vi "set_file_sent.vi"(8 "error in (no error)":errorcluster, 10 "path array in":path[](array[path]), 11 "ErrorController in":refnum<class "ErrorController.lvclass">) -> (0 "error out":errorcluster, 3 "ErrorController out":refnum<class "ErrorController.lvclass">)   [LabVIEW 2010, in "ErrorController.lvclass"]
uses:
  ErrorController.lvclass
  <vilib>/Utility/file.llb/Write To Spreadsheet File (string).vi
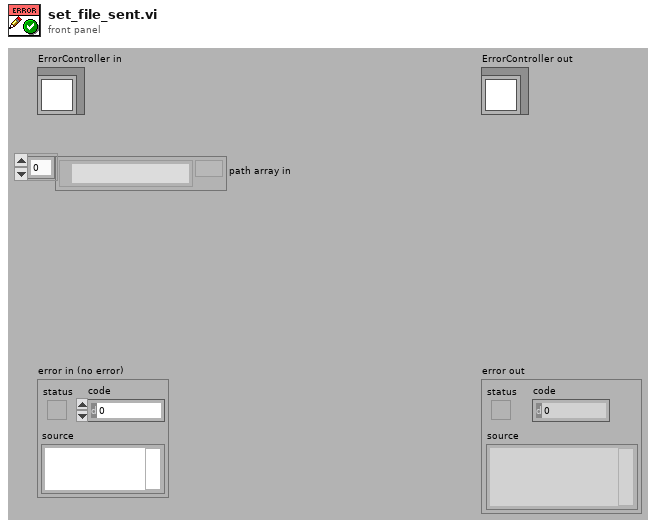
[diagram p1: front panel]
types:
  T1 = enum16{"open", "replace", "create", "open or create", "replace or create", "replace or create with confirmation"}
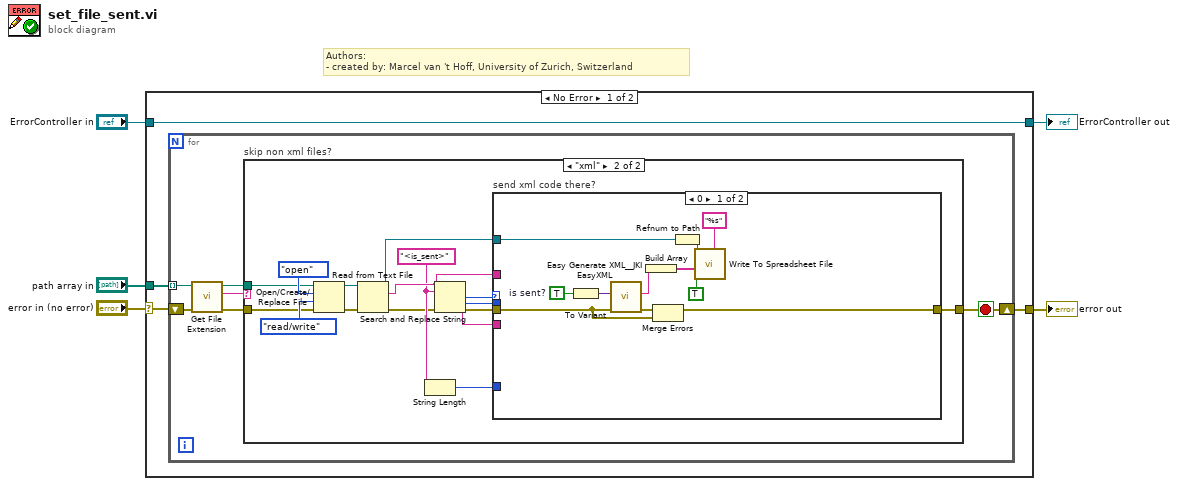
[diagram p0: block diagram]
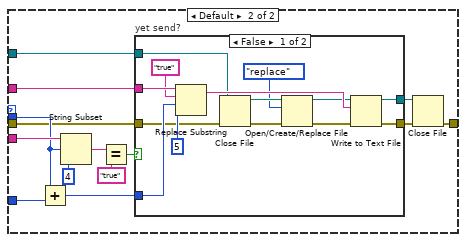
[diagram p3: hidden frame]
diagram:
  # "Authors: \n- created by: Marcel van 't Hoff, University of Zurich, Switzerland"
  n1 = case shown="No Error" "error in (no error)" {
    selector: "error in (no error)" -> [w8 w75]
    tunnel: [w7 w75] -> w4
    tunnel: [w9 w74] -> w2
    tunnel: "ErrorController in" -> [w9 w74]
    tunnel: "path array in" -> [w6 _]
    frame No Error {
      n2 = for {
        tunnel: w6 -> [w12] mode=indexing
        shift-right: [w15] -> w7
        shift-left: w8 -> [w14]
        stop <- w15 stop-if-true
        n3 = call <vilib>:"Get File Extension.vi"("error in (no error)"=w14, "file"=w12) -> ("error out"=w13:errorcluster, "lowercase file extension"=w10:string, "dup file"=w11:path)  [unwired: 6 in, 1 out]
        n4 = case "skip non xml files?" shown="\"xml\"" w10 {
          tunnel: w11 -> [_ w29]
          tunnel: w13 -> [w16 w23]
          tunnel: [w16 w19] -> w15
          frame Default {
          }
          frame "xml" {
            w26 = "<is_sent>" ("search string")
            n5 = Open/Create/Replace File(file path (use dialog)=w29, error in=w23, operation (0:open)=T1."open", access (0:read/write)=enum16{"read/write", "read-only", "write-only"}."read/write") -> (refnum out=w18:refnum<file>, error out=w30:errorcluster)  [unwired: 2 in, 1 out]
            n6 = Read from Text File(file (use dialog)=w18, error in=w30) -> (refnum out=w17:refnum<file>, text=w27:string, error out=w22:errorcluster)  [unwired: 2 in, 1 out]
            n7 = String Length(string=w26) -> (length=w25:i32)
            n8 = Search and Replace String(input string=w27, search string=w26, error in=w22) -> (result string=w28:string, number of replacements=w20:i32, offset past replacement=w24:i32, error out=w21:errorcluster)  [unwired: 5 in]
            n9 = case "send xml code there?" shown="0" w20 {
              tunnel: w28 -> [_ w53]
              tunnel: w17 -> [w37 w52]
              tunnel: w27 -> [_ w51]
              tunnel: w25 -> [_ w50]
              tunnel: w24 -> [_ w49]
              tunnel: [w33 w46] -> w19
              tunnel: w21 -> [w35 w44]
              frame 0 {
                w38 = TRUE  # is sent?
                n10 = To Variant(anything=w38) -> (Variant=w39:variant)
                n11 = call <vilib>:"Easy Generate XML__JKI EasyXML.vi"("error in (no error)"=w35, "LabVIEW Data"=w39) -> ("error out"=w34:errorcluster, "XML String"=w42:string)  [unwired: 8 in]
                n12 = Build Array(w42) -> (w43:string[])
                n13 = Merge Errors(w34, w35) -> (w33:errorcluster)
                n14 = Refnum to Path(1:w37) -> (0:w36:path)
                n15 = call-poly <vilib>:"Write To Spreadsheet File.vi"("format (%s)"="%s" ("format (%.3f)"), "append to file? (new file:F)"=TRUE, "1D data"=w43, "file path (dialog if empty)"=w36) -> ()  [unwired: 4 in, 1 out]
              }
              frame Default {
                n16 = Add(x=w49, y=w50) -> (x+y=w48:i32)
                n17 = String Subset(string=w53, offset (0)=w49, length (rest)=4 ("length (rest)")) -> (substring=w57:string)
                n18 = Equal?(x=w57, y="true") -> (x = y?=w54:bool)
                n19 = case "yet send?" shown="False" w54 {
                  tunnel: w51 -> [w69 _]
                  tunnel: w52 -> [w64 w73]
                  tunnel: w44 -> [w63 w72]
                  tunnel: [w71 w72] -> w45
                  tunnel: [w70 w73] -> w47
                  tunnel: w48 -> [w68 _]
                  frame False {
                    n20 = Replace Substring(2:5 ("length (len. of substring)"), 3:w68, 4:"true" ("replace string (\"\")"), 5:w69) -> (1:w65:string)  [unwired: 1 out]
                    n21 = Close File(refnum=w64, error in=w63) -> (path=w62:path, error out=w61:errorcluster)
                    n22 = Open/Create/Replace File(file path (use dialog)=w62, error in=w61, operation (0:open)=T1."replace") -> (refnum out=w59:refnum<file>, error out=w58:errorcluster)  [unwired: 3 in, 1 out]
                    n23 = Write to Text File(file (use dialog)=w59, text=w65, error in=w58) -> (refnum out=w70:refnum<file>, error out=w71:errorcluster)  [unwired: 1 in, 1 out]
                  }
                  frame True {
                  }
                }
                n24 = Close File(refnum=w47, error in=w45) -> (error out=w46:errorcluster)  [unwired: 1 out]
              }
            }
          }
        }
      }
    }
    frame Error {
    }
  }
  "error out" <- w4
  "ErrorController out" <- w2
